vi "View File.vi"(8 "error in":errorcluster, 11 "File in":refnum<class "File.lvclass">) -> (0 "error out":errorcluster, 3 "File out":refnum<class "File.lvclass">)   [LabVIEW 2019, in "ManejoArchivos.lvlib" / "File.lvclass"]
uses:
  File.lvclass
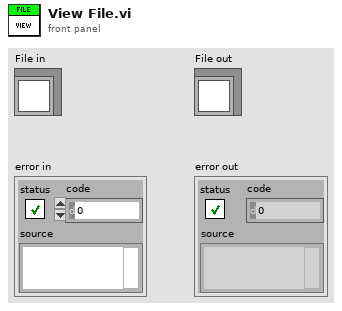
[diagram p1: front panel]
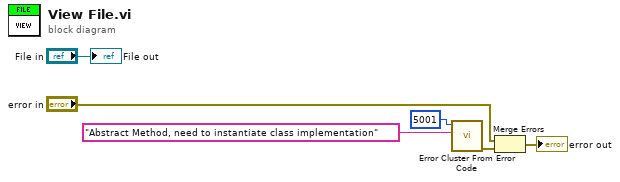
[diagram p0: block diagram]
diagram:
  n1 = call <vilib>:"Error Cluster From Error Code.vi"("error message (\"\")"="Abstract Method, need to instantiate class implementation" ("error message (\"\")"), "error code (0)"=5001) -> ("error out"=w4:errorcluster)  [unwired: 7 in]
  n2 = Merge Errors("error in", w4) -> (→"error out":errorcluster)
  "File out" <- "File in"
